vi "FRC Retroreflective Processing Example.vi"() -> ()   [LabVIEW 2014]
uses:
  <vilib>/Rock Robotics/WPI/Camera/WPI_CameraSettings Read MJPG.ctl
  <vilib>/Rock Robotics/WPI/Camera/WPI_CameraImageSize.ctl
  Vision Support Code/Camera Types.ctl
  <vilib>/vision/NI_Vision_Development_Module.lvlib
panel:
  in  "Camera Type":T1=enum."MS HD3000 square"
  in  "Image Path":path=path "Sample Images/KicoffFilmingVision"
  in  "image files":string[](array[string])
  in  "Aspect Fudge Factor":dbl=1.0
  out "Detected Totes":T2(array[cluster]) {"Normalized Rect"."Numeric 5" format="%#_2g"; "Normalized Rect"."Numeric 3" format="%#_2g"; "Normalized Rect"."Numeric 2" format="%#_2g"; "Normalized Rect"."Numeric" format="%#_2g"}
  in  "Score Threshold":dbl=75.0
  in  "Source":enum32{"Files", "Camera"}(tab)
  in  "Images":i32(listbox)
  in  "Folder Location":path=path "Sample Images/KicoffFilmingVision"
  in  "Camera Settings":T3={"fps"=20, "compression"=30, "Image Size"=enum."320x240"}
  in  "Camera Address":string="USB 1"
  in  "Annotate":bool=TRUE
  out "ms to process":u32
  out "Sorted Scores":T5(array[cluster]) {"Aspect Ratio" format="%#_3g"; "Area Score" format="%#_3g"; "X" format="%#_3g"; "Y" format="%#_3g"}
  out "Particles":i32
  in  "Ring Light Color":T6={"Hue"={101.37467765958063, 64.10933859299683}, "Sat"={88.03571428571429, 255.0}, "Val"={133.57142857142858, 255.0}} {"Hue" scale=0.0..255.0 scale format="%#_3g"}
  out "Masked":T7(plugin-control)
  out "Original Image":T7(plugin-control)
  # "Instructions:\nUse Source to select image files from a directory or use a USB or IP camera connected to your laptop.\nUse the Color of a ring light to threshold and build particles. Adjust calibration if needed.\nSmall modifications to the diagram will allow for intensity processing instead of color.\nAnnotations show the rectangle and the scores from top to bottom."
  # "Density Profile"
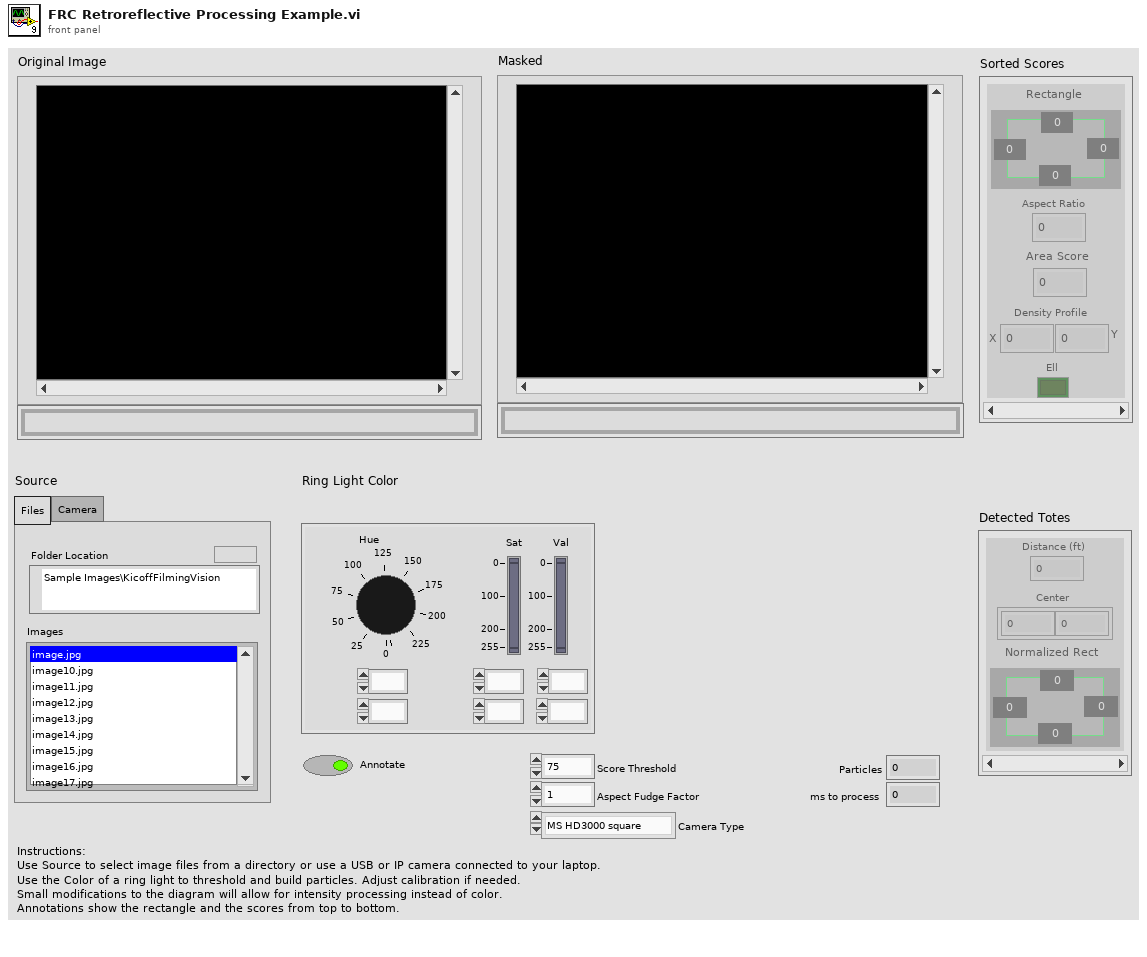
[diagram p1: front panel]
types:
  T1 = typedef "Camera Types.ctl" = enum16{"206", "1011", "1013", "MS HD3000 square", "MS HD3000 640x480"}
  T2 = cluster{"Distance (ft)":dbl, "Center":cluster{dbl, dbl}, "Normalized Rect":cluster{"Numeric":dbl, "Numeric 2":dbl, "Numeric 3":dbl, "Numeric 5":dbl}}[]
  T3 = typedef "WPI_CameraSettings Read MJPG.ctl" = cluster{"fps":i32, "compression":i32, "Image Size":T4}
  T4 = typedef "WPI_CameraImageSize.ctl" = enum16{"640x480", "320x240", "160x120", "Custom"}
  T5 = cluster{"Rectangle":cluster{"Numeric":dbl, "Numeric 2":dbl, "Numeric 3":dbl, "Numeric 5":dbl}, "Aspect Ratio":dbl, "Area Score":dbl, "X":dbl, "Y":dbl, "Ell":bool}[]
  T6 = cluster{"Hue":cluster{dbl, dbl}, "Sat":cluster{dbl, dbl}, "Val":cluster{dbl, dbl}}
  T7 = typedef "IMAQ Image.ctl" = refnum<image>
  T8 = typedef "Particle Parameters" = i32
  T9 = typedef "Image Type" = u32
  T10 = cluster{"Bounding box":cluster{"left":dbl, "top":dbl, "right":dbl, "bottom":dbl}, "Aspect Ratio":dbl, "Area Score":dbl, "X Mask":dbl, "Y Mask":dbl, "Ell":bool}[]
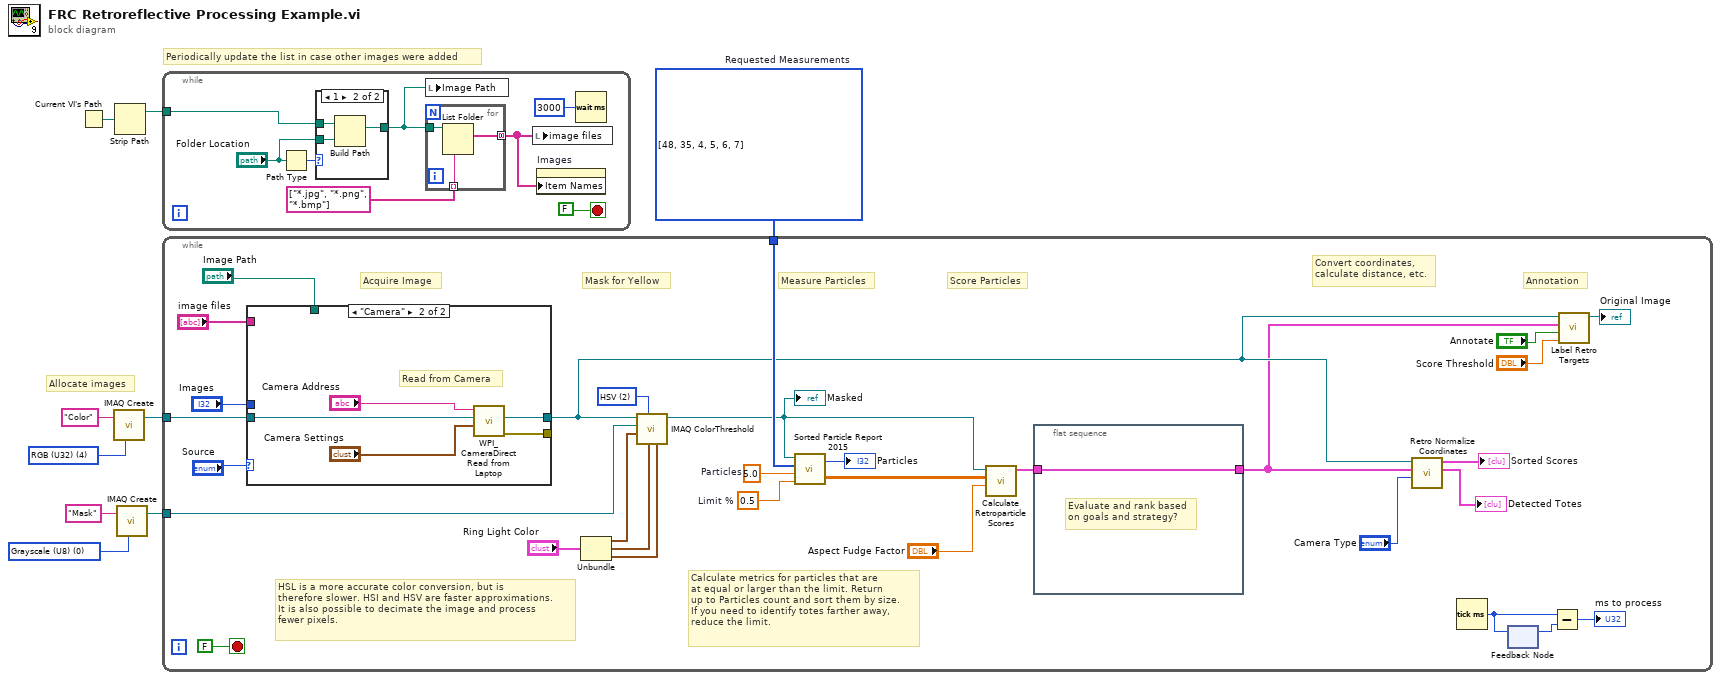
[diagram p0: block diagram]
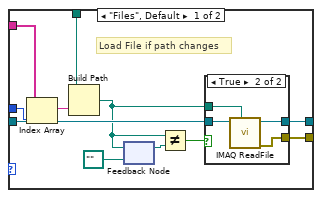
[diagram p3: hidden frame]
diagram:
  w3 = T8[] [48, 35, 4, 5, 6, 7] items=["Center of Mass X", "Center of Mass Y", "First Pixel X", "First Pixel Y", "Bounding Rect Left", "Bounding Rect Top", "Bounding Rect Right", "Bounding Rect Bottom", "Max Feret Diameter Start X", "Max Feret Diameter Start Y", "Max Feret Diameter End X", "Max Feret Diameter End Y", "Max Horiz. Segment Length Left", "Max Horiz. Segment Length Right", "Max Horiz. Segment Length Row", "-", "Bounding Rect Width", "Bounding Rect Height", "Bounding Rect Diagonal", "Perimeter", "Convex Hull Perimeter", "Holes' Perimeter", "Max Feret Diameter", "Equivalent Ellipse Major Axis", "Equivalent Ellipse Minor Axis", "Equivalent Ellipse Minor Axis (Feret)", "Equivalent Rect Long Side", "Equivalent Rect Short Side", "Equivalent Rect Diagonal", "Equivalent Rect Short Side (Feret)", "Average Horiz. Segment Length", "Average Vert. Segment Length", "Hydraulic Radius", "Waddel Disk Diameter", "-", "Area", "Holes' Area", "Particle & Holes' Area", "Convex Hull Area", "Image Area", "-", "Number of Holes", "Number of Horiz. Segments", "Number of Vert. Segments", "-", "Orientation", "Max Feret Diameter Orientation", "-", "% Area/Image Area", "% Area/(Particle & Holes' Area)", "Ratio of Equivalent Ellipse Axes", "Ratio of Equivalent Rect Sides", "-", "Elongation Factor", "Compactness Factor", "Heywood Circularity Factor", "Type Factor", "-", "Sum X", "Sum Y", "Sum XX", "Sum XY", "Sum YY", "Sum XXX", "Sum XXY", "Sum XYY", "Sum YYY", "-", "Moment of Inertia XX", "Moment of Inertia XY", "Moment of Inertia YY", "Moment of Inertia XXX", "Moment of Inertia XXY", "Moment of Inertia XYY", "Moment of Inertia YYY", "Norm. Moment of Inertia XX", "Norm. Moment of Inertia XY", "Norm. Moment of Inertia YY", "Norm. Moment of Inertia XXX", "Norm. Moment of Inertia XXY", "Norm. Moment of Inertia XYY", "Norm. Moment of Inertia YYY", "Hu Moment 1", "Hu Moment 2", "Hu Moment 3", "Hu Moment 4", "Hu Moment 5", "Hu Moment 6", "Hu Moment 7"]  # Requested Measurements
  w6 = T9 0 items=["Grayscale (U8)", "Grayscale (I16)", "Grayscale (SGL)", "Complex (CSG)", "RGB (U32)", "HSL (U32)", "RGB (U64)", "Grayscale (U16)"] ("Image Type")
  w8 = T9 4 items=["Grayscale (U8)", "Grayscale (I16)", "Grayscale (SGL)", "Complex (CSG)", "RGB (U32)", "HSL (U32)", "RGB (U64)", "Grayscale (U16)"] ("Image Type")
  # "Periodically update the list in case other images were added"
  # "Allocate images"
  n1 = Current VI's Path() -> (path=w2:path)
  n2 = call "IMAQ Create"("Image Name"="Color", "Image Type"=w8) -> ("New Image"=w7:T7)  [unwired: 2 in, 2 out]
  n3 = Strip Path(path=w2) -> (stripped path=w1:path)  [unwired: 1 out]
  n4 = call "IMAQ Create"("Image Name"="Mask", "Image Type"=w6) -> ("New Image"=w4:T7)  [unwired: 2 in, 2 out]
  n5 = while {
    tunnel: w1 -> [w11]
    stop <- FALSE stop-if-true
    n6 = Path Type(1:"Folder Location") -> (0:w13:i16)
    n7 = case shown="1" w13 {
      tunnel: "Folder Location" -> [w18 w21]
      tunnel: [w18 w19] -> w10
      tunnel: w11 -> [_ w20]
      frame 0, Default {
      }
      frame 1 {
        n8 = Build Path(base path=w20, name or relative path=w21) -> (appended path=w19:path)
      }
    }
    n9 = local write "Image Path"(w10) -> ()
    n10 = for {
      tunnel: [w24] -> w14 mode=concatenating
      tunnel: w10 -> [w23]
      tunnel: string[] ["*.jpg", "*.png", "*.bmp"] -> [w22] mode=indexing
      n11 = List Folder(path=w23, pattern=w22) -> (filenames=w24:string[])  [unwired: 2 in, 3 out]
    }
    n12 = local write "image files"(w14) -> ()
    n13 = property on="Images" class="LstBox (strict)"("Item Names"=w14) -> ()  [unwired: 2 in, 2 out]
    n14 = Wait (ms)(milliseconds to wait=u32 3000) -> ()  [unwired: 1 out]
  }
  n15 = while {
    tunnel: w7 -> [w54]
    tunnel: w4 -> [w52]
    tunnel: w3 -> [w46]
    stop <- FALSE stop-if-true
    w43 = 0.5  # Limit %
    w45 = 5.0  # Particles
    w51 = u16 2 items=["RGB", "HSL", "HSV", "HSI"] ("Color Mode")
    # "Calculate metrics for particles that are\nat equal or larger than the limit. Return\nup to Particles count and sort them by size.\nIf you need to identify totes farther away,\nreduce the limit."
    # "Measure Particles"
    # "Convert coordinates,\ncalculate distance, etc."
    # "Annotation"
    # "Score Particles"
    # "Mask for Yellow"
    # "Acquire Image"
    # "HSL is a more accurate color conversion, but is\ntherefore slower. HSI and HSV are faster approximations.\nIt is also possible to decimate the image and process\nfewer pixels."
    n16 = case shown="\"Camera\"" "Source" {
      tunnel: [w66 w77] -> _
      tunnel: [w67 w76] -> w31
      tunnel: w54 -> [w65 w75]
      tunnel: "image files" -> [w57 _]
      tunnel: "Images" -> [w64 _]
      tunnel: "Image Path" -> [w62 _]
      frame "Files", Default {
        # "Load File if path changes"
        n17 = Index Array(array=w57, index=w64) -> (element=w63:string)
        n18 = Build Path(base path=w62, name or relative path=w63) -> (appended path=w58:path)
        n19 = feedback-in #1(w58) -> ()
        n20 = feedback #1(path "" ("appended path")) -> (w60:path)
        n21 = Not Equal?(x=w58, y=w60) -> (x != y?=w61:bool)
        n22 = case shown="True" w61 {
          tunnel: [w68 w72] -> w67
          tunnel: [_ w71] -> w66
          tunnel: w65 -> [w68 w70]
          tunnel: w58 -> [_ w69]
          frame False {
          }
          frame True {
            n23 = call "IMAQ ReadFile"("File Path"=w69, "Image"=w70) -> ("error out"=w71:errorcluster, "Image Out"=w72:T7)  [unwired: 5 in, 3 out]
          }
        }
      }
      frame "Camera" {
        # "Read from Camera"
        n24 = call <vilib>:"WPI_CameraDirect Read from Laptop.vi"("Camera Settings"="Camera Settings", "Image"=w75, "address"="Camera Address") -> ("error out"=w77:errorcluster, "Image Out"=w76:T7)  [unwired: 7 in]
      }
    }
    n25 = Unbundle("Ring Light Color") -> ("Hue"=w50:cluster{dbl, dbl}, "Sat"=w49:cluster{dbl, dbl}, "Val"=w48:cluster{dbl, dbl})
    n26 = call "IMAQ ColorThreshold"("Blue or Luma or Val or Inten Range"=w48, "Green or Sat Range"=w49, "Color Mode"=w51, "Red or Hue Range"=w50, "Image Dst"=w52, "Image Src"=w31) -> ("Image Dst Out"=w36:T7)  [unwired: 4 in, 1 out]
    "Masked" <- w36
    n27 = call "Sorted Particle Report 2015.vi"("Min Area Size %"=w43, "Particle Count Limit"=w45, "Pixel Measurements"=w46, "Image in"=w36) -> ("Sorted Data"=w33:dbl[][], "Particles"=→"Particles":i32)
    n28 = call "Calculate Retroparticle Scores.vi"("Aspect Fudge Factor"="Aspect Fudge Factor", "Sorted Data"=w33, "Image in"=w36) -> ("Scores"=w35:T10)  [unwired: 8 in]
    n29 = flat-sequence {
      tunnel: w35 -> [w56]
      tunnel: [w56] -> w28
      frame #0 {
        # "Evaluate and rank based\non goals and strategy?"
      }
    }
    n30 = call "Retro Normalize Coordinates.vi"("Camera Type"="Camera Type", "Scores"=w28, "Image in"=w31) -> ("Found Totes"=→"Detected Totes":T2, "Sorted Scores"=→"Sorted Scores":T5)  [unwired: 7 in]
    n31 = Tick Count (ms)() -> (millisecond timer value=w41:u32)
    n32 = feedback-in #2(w41) -> ()
    n33 = feedback #2() -> (w42:u32)  [unwired: 1 in]
    n34 = Subtract(x=w41, y=w42) -> (x-y=→"ms to process":u32)
    n35 = call "Label Retro Targets.vi"("Score Threshold"="Score Threshold", "Annotate"="Annotate", "Scores"=w28, "Image in"=w31) -> ("Image out"=→"Original Image":T7)  [unwired: 7 in]
  }
